vi "New.vi"(8 "error in (no error)":errorcluster, 9 "remote port or service name":u16=7776, 10 "address":string="192.168.24.142") -> (0 "error out":errorcluster, 3 "Lifter_motor out":refnum<class "Lifter_motor.lvclass">)   [LabVIEW 2019, in "Lifter_motor.lvclass"]
uses:
  Lifter_motor.lvclass
  Lifter_motor.lvclass/Lifter_motor.ctl
  TCP Class/LifterTCP.lvclass
panel:
  in  "Roots(For backlash)":bool
  in  "Lifter_motor in":refnum<class "Lifter_motor.lvclass">
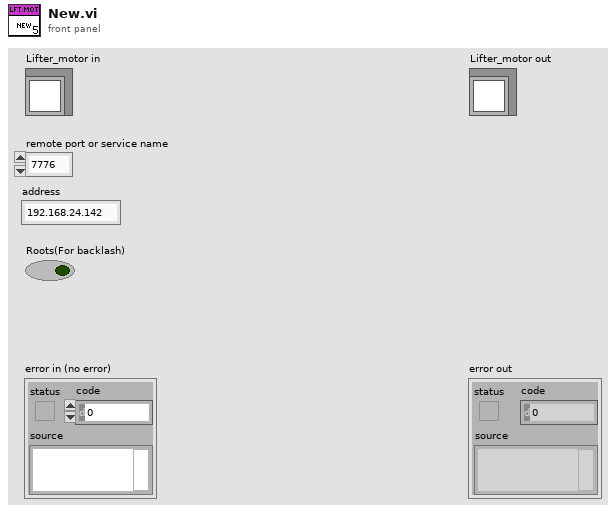
[diagram p1: front panel]
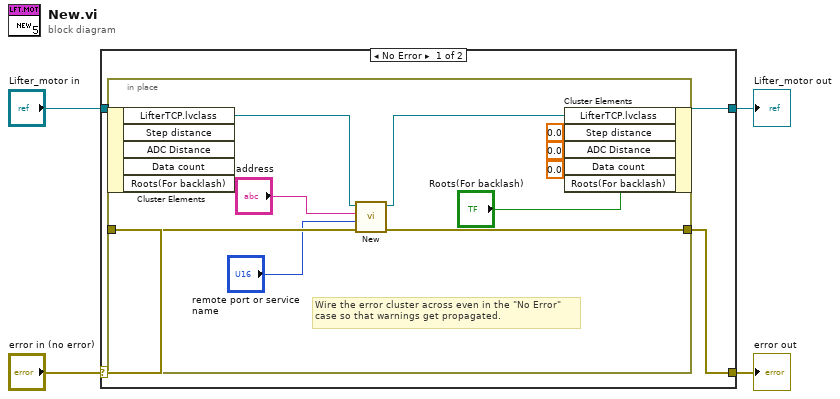
[diagram p0: block diagram]
diagram:
  n1 = case shown="No Error" "error in (no error)" {
    selector: "error in (no error)" -> [w6 w20]
    tunnel: [w5 w20] -> w3
    tunnel: [w7 w19] -> w1
    tunnel: "Lifter_motor in" -> [w8 w19]
    frame No Error {
      n2 = in-place {
        in-place-border: w6 -> [w16]
        in-place-border: [w15] -> w5
        # "Wire the error cluster across even in the \"No Error\"\ncase so that warnings get propagated."
        n3 = in-place-cluster #1(w8) -> ("LifterTCP.lvclass"=w18:refnum<class "LifterTCP.lvclass">)  [unwired: 4 out]
        n4 = call "New.vi"("error in (no error)"=w16, "remote port or service name"="remote port or service name", "address"="address", "LifterTCP in"=w18) -> ("error out"=w15:errorcluster, "LifterTCP out"=w17:refnum<class "LifterTCP.lvclass">)  [unwired: 6 in]
        n5 = in-place-cluster #1("LifterTCP.lvclass"=w17, "Step distance"=0.0, "ADC Distance"=0.0, "Data count"=0.0, "Roots(For backlash)"="Roots(For backlash)") -> (w7:refnum<class "Lifter_motor.lvclass">)
      }
    }
    frame Error {
    }
  }
  "error out" <- w3
  "Lifter_motor out" <- w1
